vi "Send To Creator.vi"(4 "Is Priority":bool, 7 "Actor in":refnum<class "Actor.lvclass">, 9 "Error":errorcluster, 10 "Actor":refnum<class "Actor.lvclass">) -> (0 "Error out":errorcluster)   [LabVIEW 2025, in "jettl.lvlib" / "Finish Msg.lvlib"]
uses:
  Finish Msg.lvlib
  Actor/Actor/Actor.lvclass
  Finish Msg/Finish Msg.lvclass
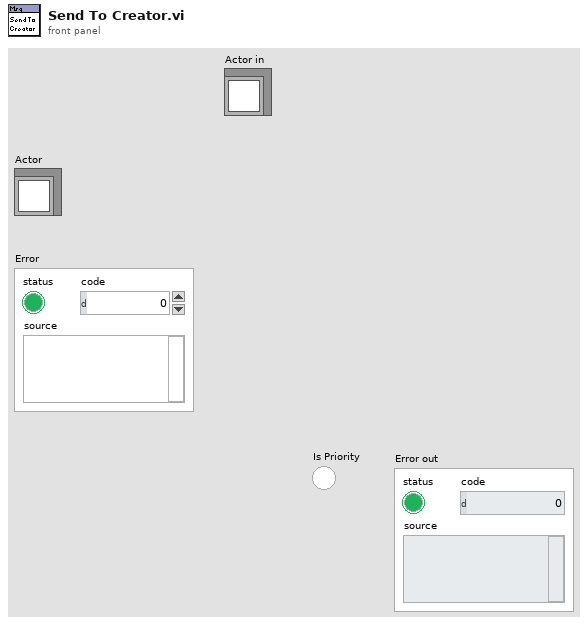
[diagram p1: front panel]
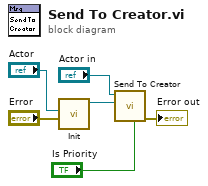
[diagram p0: block diagram]
diagram:
  n1 = call "Init.vi"("Error"="Error", "Actor"="Actor") -> ("Finish Msg out"=w3:refnum<class "Finish Msg.lvclass">)  [unwired: 9 in]
  n2 = call-dynamic "Send To Creator.vi"("Is Priority"="Is Priority", "Msg"=w3, "Actor in"="Actor in") -> ("Error out"=→"Error out":errorcluster)  [unwired: 8 in]
